vi "FPGA_Interface_Create.vi"(0 "reference in":refnum<class "FPGA_Interface.lvclass">, 11 "error in (no error)":errorcluster) -> (4 "reference out":refnum<class "FPGA_Interface.lvclass">, 15 "error out":errorcluster)   [LabVIEW 2019]
doc: "Constructor."
uses:
  <vilib>/addons/_AddQ/G#Object/G#Object.lvclass
  FPGA_Interface.lvclass
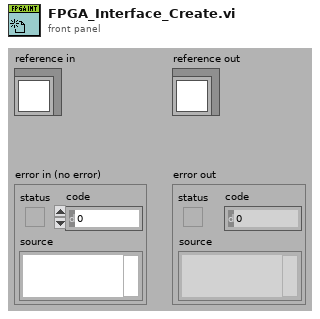
[diagram p1: front panel]
types:
  T1 = typedef "FPGA_Interface.lvclass/ObjectAttributesRef.ctl" = refnum<data-value>
  T2 = typedef "FPGA_Interface.lvclass/ObjectAttributes.ctl" = cluster{"MyAttribute":dbl}
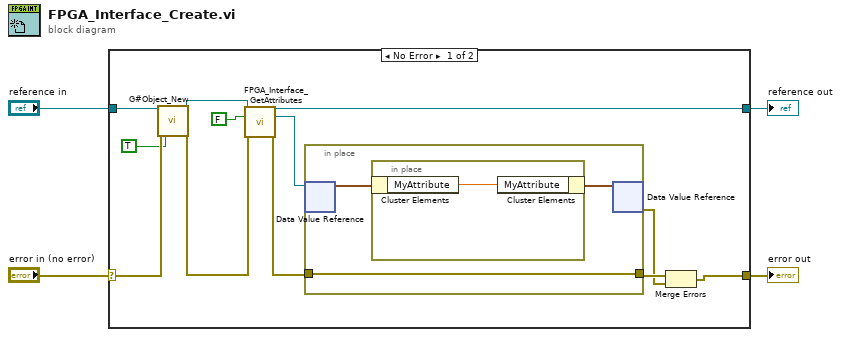
[diagram p0: block diagram]
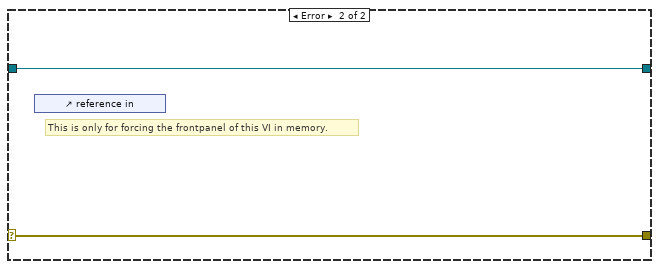
[diagram p2: hidden frame]
diagram:
  n1 = case shown="No Error" "error in (no error)" {
    selector: "error in (no error)" -> [w15 w22]
    tunnel: [w14 w22] -> w3
    tunnel: [w9 w21] -> w1
    tunnel: "reference in" -> [w16 w21]
    frame No Error {
      n2 = call <vilib>:"G#Object_New.vi"("reference in"=w16, "error in (no error)"=w15, "user counter (T)?"=TRUE ("User Counter")) -> ("reference out"=w10:refnum<class "G#Object.lvclass">, "error out"=w8:errorcluster)  [unwired: 14 in, 1 out]
      n3 = call "FPGA_Interface_GetAttributes.vi"("reference in"=w10, "return data? (T)"=FALSE ("return data"), "error in (no error)"=w8) -> ("reference out"=w9:refnum<class "FPGA_Interface.lvclass">, "attributes ref"=w6:T1, "error out"=w7:errorcluster)  [unwired: 9 in, 1 out]
      n4 = in-place {
        in-place-border: w7 -> [w17]
        in-place-border: [w17] -> w12
        n5 = in-place-dvr #1(w6) -> (w18:T2)  [unwired: 1 out]
        n6 = in-place {
          n7 = in-place-cluster #2(w18) -> ("MyAttribute"=w20:dbl)
          n8 = in-place-cluster #2("MyAttribute"=w20) -> (w19:T2)
        }
        n9 = in-place-dvr #1(w19) -> (w11:errorcluster)  [unwired: 1 out]
      }
      n10 = Merge Errors(w12, w11) -> (w14:errorcluster)
    }
    frame Error {
      # "This is only for forcing the frontpanel of this VI in memory."
      n11 = control-ref of="reference in"() -> ()  [unwired: 1 out]
    }
  }
  "error out" <- w3
  "reference out" <- w1
